vi "logica_sube_baja.vi"(0 "Baja A":bool, 3 "Baja B":bool, 4 "Sube B":bool, 5 "Sube A":bool) -> (1 "Numeric":i32, 2 "Numeric 2":i32)   [LabVIEW 2021]
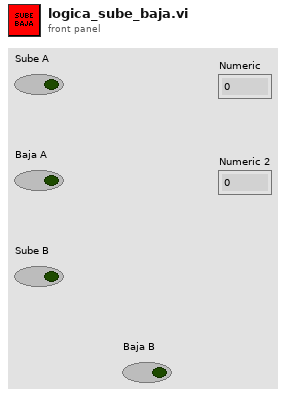
[diagram p1: front panel]
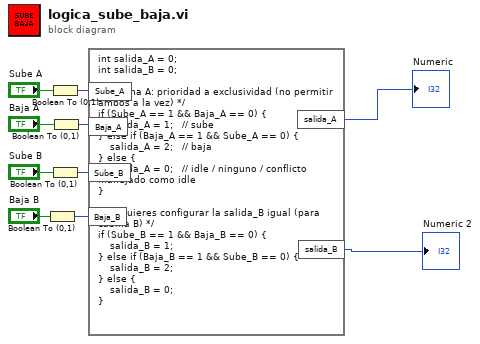
[diagram p0: block diagram]
diagram:
  n1 = Boolean To (0,1)(Boolean="Baja B") -> (0, 1=w1:i16)
  n2 = Boolean To (0,1)(Boolean="Sube A") -> (0, 1=w2:i16)
  n3 = Boolean To (0,1)(Boolean="Sube B") -> (0, 1=w4:i16)
  n4 = Boolean To (0,1)(Boolean="Baja A") -> (0, 1=w3:i16)
  n5 = formula code="int salida_A = 0;\nint salida_B = 0;\n\n/* Cabina A: prioridad a exclusividad (no permitir ambos a la vez) */\nif (Sube_A == 1 && Baja_A == 0) {\n    salida_A = 1;   // sube\n} else if (Baja_A == 1 && Sube_A == 0) {\n    salida_A = 2;   // baja\n} else {\n    salida_A = 0;   // idle / ninguno / conflicto manejado como idle\n}\n\n/* Si quieres configurar la salida_B igual (para cabina B) */\nif (Sube_B == 1 && Baja_B == 0) {\n    salida_B = 1;\n} else if (Baja_B == 1 && Sube_B == 0) {\n    salida_B = 2;\n} else {\n    salida_B = 0;\n}"("Sube_A"=w2, "Baja_A"=w3, "Sube_B"=w4, "Baja_B"=w1) -> ("salida_A"=→"Numeric":i32, "salida_B"=→"Numeric 2":i32)
